vi "StatusBar.vi"() -> ()   [LabVIEW 2020]
panel:
  out "String 2":string
  out "String":string
  in  "stop":bool
  in  "B":bool
  in  "A":bool
  # "Decoration boxes"
  # "String Indicators sized to fit in decoration box"
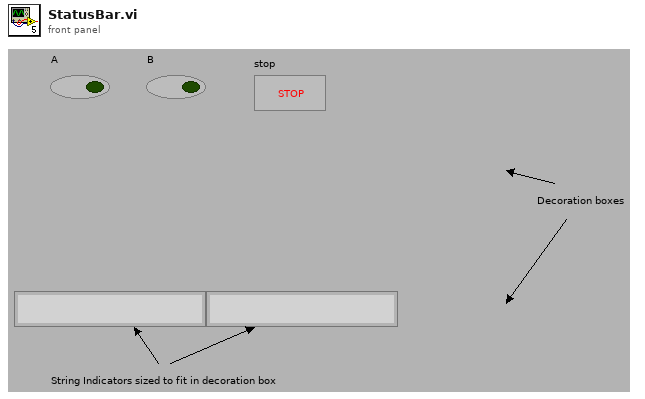
[diagram p1: front panel]
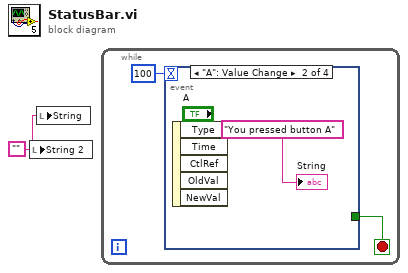
[diagram p0: block diagram]
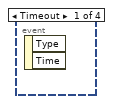
[diagram p2: hidden frame]
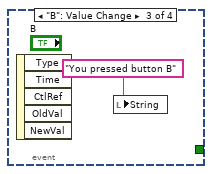
[diagram p3: hidden frame]
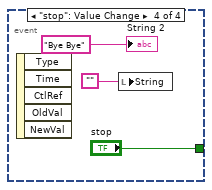
[diagram p4: hidden frame]
diagram:
  w1 = ""
  n1 = local write "String 2"(w1) -> ()
  n2 = local write "String"(w1) -> ()
  n3 = while {
    stop <- w2 stop-if-true
    n4 = event shown="[1] \"A\": Value Change" {
      selector: _ -> [_ _ _ _]
      dyn-events: _ -> [_ _ _ _]
      timeout: 100 -> [_ _ _ _]
      tunnel: [_ _ _ "stop"] -> w2
      event Timeout {
        n5 = event-data() -> ()  [unwired: 1 in, 2 out]
      }
      event "A": Value Change {
        n6 = event-data() -> ()  [unwired: 1 in, 5 out]
        "String" <- "You pressed button A"
      }
      event "B": Value Change {
        n7 = event-data() -> ()  [unwired: 1 in, 5 out]
        n8 = local write "String"("You pressed button B") -> ()
      }
      event "stop": Value Change {
        n9 = event-data() -> ()  [unwired: 1 in, 5 out]
        n10 = local write "String"("") -> ()
        "String 2" <- "Bye Bye"
      }
    }
  }
